vi "8avgU8.vi"(11 "input":u8) -> (3 "output":u8)   [LabVIEW 2010, in "KevLib01.lvlib"]
uses:
  KevLib01.lvlib
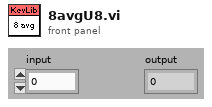
[diagram p1: front panel]
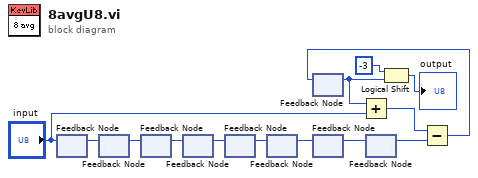
[diagram p0: block diagram]
diagram:
  n1 = feedback-in #1("input") -> ()
  n2 = feedback #1() -> (w1:u8)  [unwired: 1 out]
  n3 = feedback-in #2(w1) -> ()
  n4 = feedback #2() -> (w2:u8)  [unwired: 1 out]
  n5 = feedback-in #3(w2) -> ()
  n6 = feedback #3() -> (w3:u8)  [unwired: 1 out]
  n7 = feedback-in #4(w3) -> ()
  n8 = feedback #4() -> (w4:u8)  [unwired: 1 out]
  n9 = feedback-in #5(w4) -> ()
  n10 = feedback #5() -> (w5:u8)  [unwired: 1 out]
  n11 = feedback-in #6(w5) -> ()
  n12 = feedback #6() -> (w6:u8)  [unwired: 1 out]
  n13 = feedback #7() -> (w11:u8)  [unwired: 1 out]
  n14 = feedback-in #8(w6) -> ()
  n15 = feedback #8() -> (w9:u8)  [unwired: 1 out]
  n16 = Add(x=w11, y="input") -> (x+y=w7:u8)
  n17 = feedback-in #9(w9) -> ()
  n18 = feedback #9() -> (w10:u8)  [unwired: 1 out]
  n19 = Logical Shift(y=i8 -3, x=w11) -> (x << y=→"output":u8)
  n20 = Subtract(x=w7, y=w10) -> (x-y=w8:u8)
  n21 = feedback-in #7(w8) -> ()
